vi "set serial number.vi"(8 "error in (no error)":errorcluster, 10 "serial_number":T1, 11 "id":i32) -> (0 "error out":errorcluster, 3 "function return":i32)   [LabVIEW 2012, in "libximc.lvlib"]
doc: "result_t XIMC_API set_serial_number (device_t id, const serial_number_t* serial_number);"
uses:
  libximc.lvlib
  libximc.dll
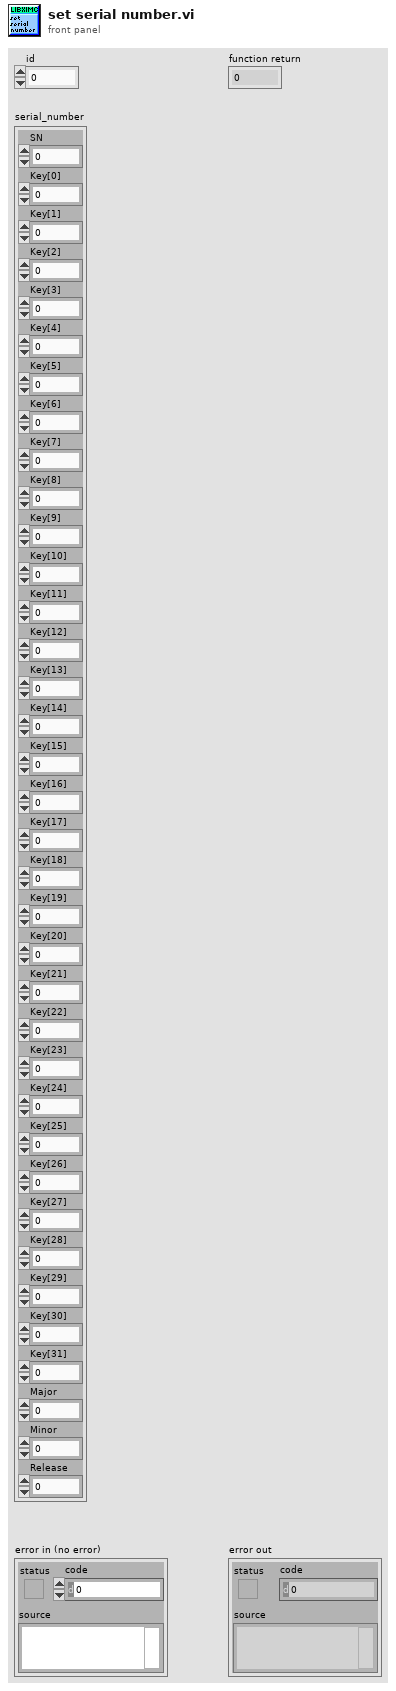
[diagram p1: front panel]
types:
  T1 = cluster{"SN":u32, "Key[0]":u8, "Key[1]":u8, "Key[2]":u8, "Key[3]":u8, "Key[4]":u8, "Key[5]":u8, "Key[6]":u8, "Key[7]":u8, "Key[8]":u8, "Key[9]":u8, "Key[10]":u8, "Key[11]":u8, "Key[12]":u8, "Key[13]":u8, "Key[14]":u8, "Key[15]":u8, "Key[16]":u8, "Key[17]":u8, "Key[18]":u8, "Key[19]":u8, "Key[20]":u8, "Key[21]":u8, "Key[22]":u8, "Key[23]":u8, "Key[24]":u8, "Key[25]":u8, "Key[26]":u8, "Key[27]":u8, "Key[28]":u8, "Key[29]":u8, "Key[30]":u8, "Key[31]":u8, "Major":u32, "Minor":u32, "Release":u32}
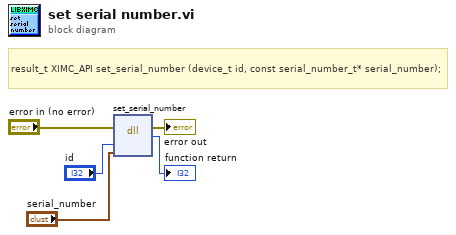
[diagram p0: block diagram]
diagram:
  # "result_t XIMC_API set_serial_number (device_t id, const serial_number_t* serial_number);"
  n1 = dll-call lib="C:/Users/user/Desktop/labview-2.9.11-gen/libximc.*" fn="set_serial_number"(error in="error in (no error)", "id"="id", "serial_number"="serial_number") -> (error out=→"error out":errorcluster, →"function return":i32)  [unwired: 4 in, 1 out]
